vi "Tell Self.vi"(4 "Priority":bool, 7 "Actor in":refnum<class "Actor.lvclass">) -> (0 "Error out":errorcluster)   [LabVIEW 2025, in "_Template.lvlib" / "Templates.lvlib" / "TEMPLATE jettl Msg.lvlib"]
uses:
  TEMPLATE jettl Msg.lvlib
  jettl/jettl/Actor/Actor.lvclass
  Init Msg.vi
  jettl/jettl/jettl.lvlib
panel:
  # "This front panel should not be manipulated."
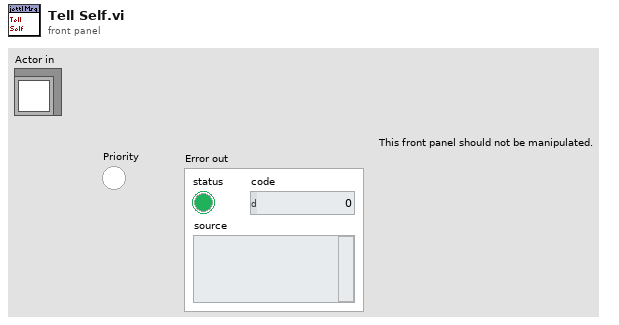
[diagram p1: front panel]
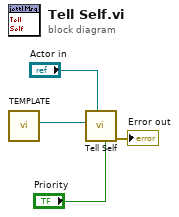
[diagram p0: block diagram]
diagram:
  n1 = call-poly "TEMPLATE.vi"() -> ("Msg"=w1:refnum<class "Msg.lvclass">)  [unwired: 11 in]
  n2 = call "Tell Self.vi"("Priority"="Priority", "Actor in"="Actor in", "Msg"=w1) -> ("Error out"=→"Error out":errorcluster)  [unwired: 8 in]
